vi "SVT Weighting Filter (N Ch).vi"(5 "reset filter (F)":bool, 7 "error in (no error)":errorcluster, 9 "weighting":u16(ring) items=["Linear", "A-weighting", "B-weighting", "C-weighting"], 10 "scaled signals [EU]":waveform(dbl)[](array[waveform])) -> (0 "error out":errorcluster, 3 "weighted signals [EU]":waveform(dbl)[](array[waveform]))   [LabVIEW 2017, in "SoundVib_ABCWeighting.lvlib"]
doc: "Applies the selected weighting to <B>scaled signal [EU]</B>. This VI complies with ANSI S1.4-1983, ANSI S1.42-2001, IEC 61672-1:2002, and JIS C 1509-1:2005 standards. Use Each instance of this VI maintains its own state; use the N Channel instance of this VI to process an array of channels. This VI operates on time-continuous data; it resets on a discontinuity. Wire data to the <B>scaled signal [EU]</B> input to determine the polymorphic instance to use or manually select the instance."
uses:
  <vilib>/addons/Sound and Vibration/svt_Weighting/SoundVib_ABCWeighting.lvlib
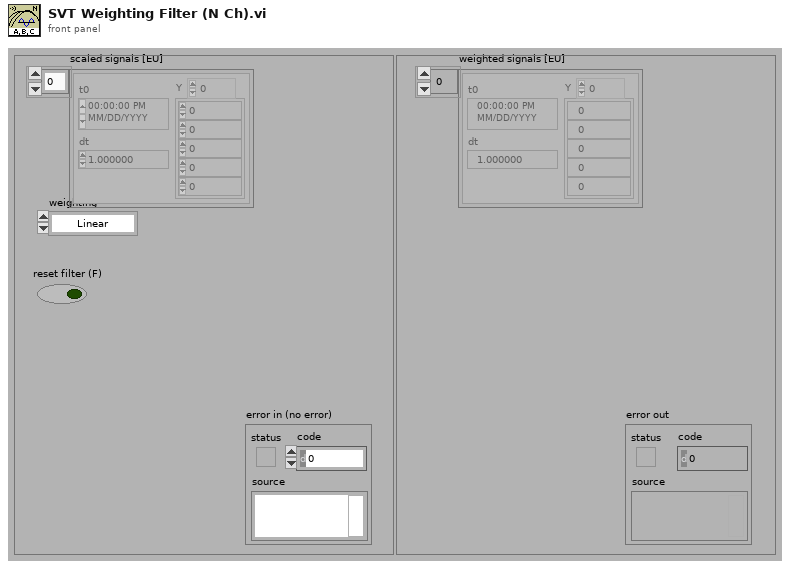
[diagram p1: front panel]
types:
  T1 = typedef "svc_Weighting Filter Text Ring.ctl" = u16
  T2 = cluster{"filter structure":enum32{"IIR 2nd Order", "IIR 4th Order"}, "Reverse Coefficients":dbl[], "Forward Coefficients":dbl[]}
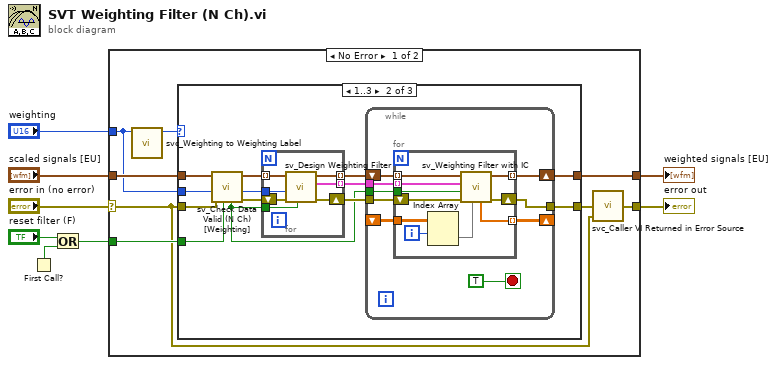
[diagram p0: block diagram]
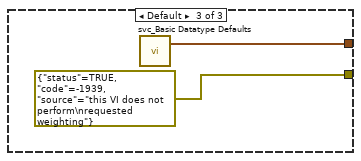
[diagram p3: hidden frame]
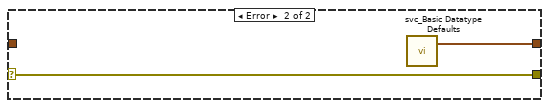
[diagram p4: hidden frame]
diagram:
  n1 = First Call?() -> (First Call?: T/F=w7:bool)
  n2 = Or(x="reset filter (F)", y=w7) -> (x .or. y?=w3:bool)
  n3 = case shown="No Error" "error in (no error)" {
    selector: "error in (no error)" -> [w9 w61]
    tunnel: "scaled signals [EU]" -> [w16 _]
    tunnel: [w12 w61] -> w5
    tunnel: [w14 w60] -> w4
    tunnel: w3 -> [w13 _]
    tunnel: "weighting" -> [w11 _]
    frame No Error {
      n4 = call <vilib>:"svc_Weighting to Weighting Label.vi"("weighting filter"=w11) -> ("weighting enum"=w10:T1)  [unwired: 9 in, 1 out]
      n5 = case shown="1..3" w10 {
        tunnel: w9 -> [w17 w27 _]
        tunnel: w16 -> [w18 w31 _]
        tunnel: [w17 w30 errorcluster {"status"=TRUE, "code"=-1939, "source"="this VI does not perform\nrequested weighting"} ("error out")] -> w15
        tunnel: [w18 w29 w59] -> w14
        tunnel: w13 -> [_ w28 _]
        tunnel: w11 -> [_ w26 _]
        frame 0 {
        }
        frame 1..3 {
          n6 = call <vilib>:"sv_Check Data Valid (N Ch) [Weighting].vi"("reset (in)"=w28, "error in (no error)"=w27, "weighting"=w26, "scaled signal [in]"=w31) -> ("error out"=w23:errorcluster, "weighting"=w20:T1, "scaled signal [out]"=w24:waveform(dbl)[], "reset (out)"=w19:bool)  [unwired: 4 in]
          n7 = for {
            tunnel: w24 -> [w38] mode=indexing
            tunnel: w20 -> [w33]
            tunnel: [w36] -> w21 mode=indexing
            tunnel: [w34] -> w25 mode=indexing
            tunnel: w19 -> [w32]
            shift-right: [w35] -> w22
            shift-left: w23 -> [w37]
            n8 = call <vilib>:"sv_Design Weighting Filter.vi"("reset filter (F)"=w32, "error in (no error)"=w37, "weighting"=w33, "scaled signal"=w38) -> ("error out"=w35:errorcluster, "filter coefficients"=w34:T2, "dup scaled signal"=w36:waveform(dbl))  [unwired: 5 in]
          }
          n9 = while {
            tunnel: w19 -> [w43]
            tunnel: [w44] -> w30
            shift-left: _ -> [w39]
            shift-right: [w47] -> _
            tunnel: w22 -> [w40]
            tunnel: w25 -> [w41]
            shift-right: [w45] -> w29
            shift-left: w21 -> [w42]
            stop <- TRUE stop-if-true
            n10 = for {
              tunnel: w39 -> [w57]
              tunnel: [w56] -> w47 mode=indexing
              tunnel: w42 -> [w55] mode=indexing
              tunnel: w41 -> [w53] mode=indexing
              tunnel: [w51] -> w45 mode=indexing
              tunnel: w43 -> [w50]
              shift-right: [w52] -> w44
              shift-left: w40 -> [w54]
              i -> [w48]
              n11 = Index Array(array=w57, index (row)=w48) -> (element=w49:dbl[])  [unwired: 1 in]
              n12 = call <vilib>:"sv_Weighting Filter with IC.vi"("Initial Filter State"=w49, "error in (no error)"=w54, "reset filter (F)"=w50, "filter coefficients"=w53, "signal [V]"=w55) -> ("error out"=w52:errorcluster, "filtered signal [EU]"=w51:waveform(dbl), "Final Filter State"=w56:dbl[])  [unwired: 4 in]
            }
          }
        }
        frame Default {
          n13 = call <vilib>:"svc_Basic Datatype Defaults.vi"() -> ("empty array of waveforms"=w59:waveform(dbl)[])  [unwired: 7 in, 12 out]
        }
      }
      n14 = call <vilib>:"svc_Caller VI Returned in Error Source.vi"("warning input to caller"=w9, "error in (no error)"=w15) -> ("error out"=w12:errorcluster)  [unwired: 3 in]
    }
    frame Error {
      n15 = call <vilib>:"svc_Basic Datatype Defaults.vi"() -> ("empty array of waveforms"=w60:waveform(dbl)[])  [unwired: 7 in, 12 out]
    }
  }
  "weighted signals [EU]" <- w4
  "error out" <- w5
